vi "Clear HWI.vi"(8 "error in (no error)":errorcluster, 11 "Pulseblaster in":refnum<class "Pulseblaster.lvclass">) -> (0 "error out":errorcluster, 3 "Pulseblaster out":refnum<class "Pulseblaster.lvclass">)   [LabVIEW 2013, in "Pulseblaster.lvclass"]
uses:
  Pulseblaster.lvclass
  Pulseblaster.lvclass/Pulseblaster.ctl
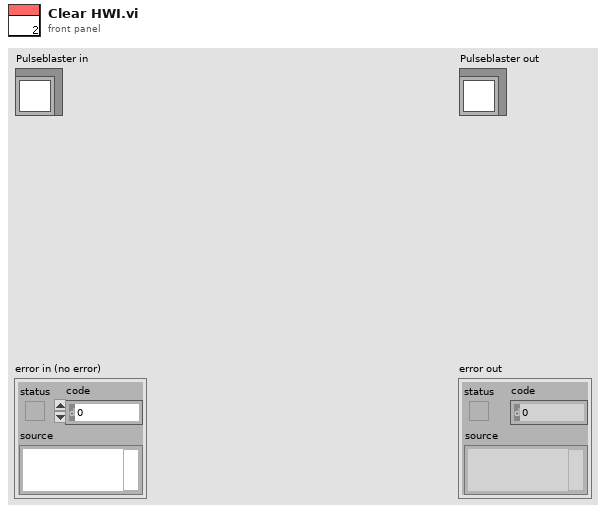
[diagram p1: front panel]
types:
  T1 = cluster{"Triggering":bool[][], "Ramp Info":cluster{"Ramp Index":i32, "Ramp Time":dbl, "Number of Steps":i32}[], "VLIW Array":cluster{"Output Bits":u32, "Data Field":u32, "OP Code":u8, "Delay Count":u64}[]}
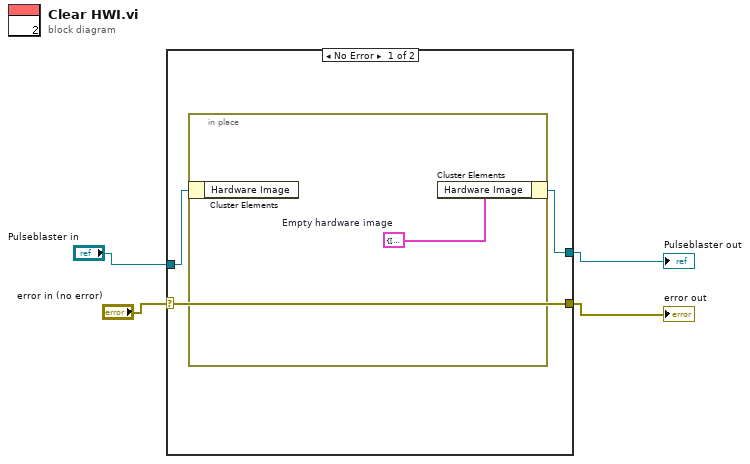
[diagram p0: block diagram]
diagram:
  n1 = case shown="No Error" "error in (no error)" {
    selector: "error in (no error)" -> [w7 w10]
    tunnel: [w7 w10] -> w2
    tunnel: [w6 w9] -> w1
    tunnel: "Pulseblaster in" -> [w5 w9]
    frame No Error {
      n2 = in-place {
        w8 = T1 {"Triggering"=[], "Ramp Info"=[], "VLIW Array"=[]}  # Empty hardware image
        n3 = in-place-cluster #1(w5) -> ()  [unwired: 1 out]
        n4 = in-place-cluster #1("Hardware Image"=w8) -> (w6:refnum<class "Pulseblaster.lvclass">)
      }
    }
    frame Error {
    }
  }
  "error out" <- w2
  "Pulseblaster out" <- w1
